vi "Hide Front Panel.vi"(8 "error in (no error)":errorcluster, 11 "Hide IA Front Panel?":bool) -> (0 "error out":errorcluster)   [LabVIEW 2020]
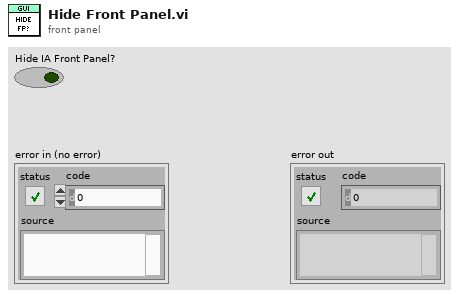
[diagram p1: front panel]
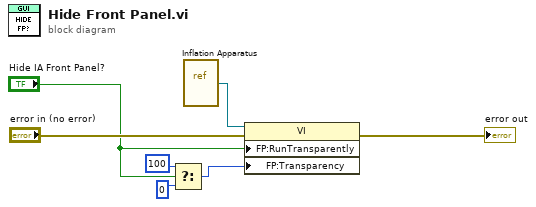
[diagram p0: block diagram]
diagram:
  n1 = Select(t=u8 100, s="Hide IA Front Panel?", f=u8 0 ("Front Panel Window:Transparency")) -> (s? t:f=w1:u8)
  n2 = vi-ref "Inflation Apparatus.vi"() -> (w5:refnum<vi>)
  n3 = property class="VI"(reference=w5, error in="error in (no error)", "FP:RunTransparently"="Hide IA Front Panel?", "FP:Transparency"=w1) -> (error out=→"error out":errorcluster)  [unwired: 1 out]
